vi "TupnOff.vi"(8 "error in (no error)":errorcluster, 11 "Pump_1AI_1DO_2DI in":refnum<class "PM_Group.lvclass">) -> (0 "error out":errorcluster, 3 "Pump_1AI_1DO_2DI out":refnum<class "PM_Group.lvclass">)   [LabVIEW 2019, in "PM_Group.lvclass"]
uses:
  PM_Group.lvclass
  TypeDef/StatePump.ctl
  FPGA_API_class/FPGA API.lvclass
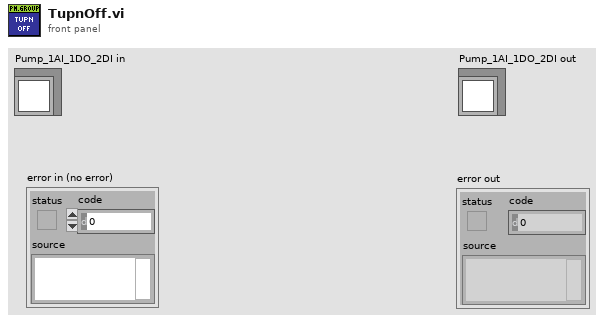
[diagram p1: front panel]
types:
  T1 = typedef "StatePump.ctl" = enum16{"Off", "TupningOn", "On", "TurningOff"}
  T2 = typedef "DO index.ctl" = u8
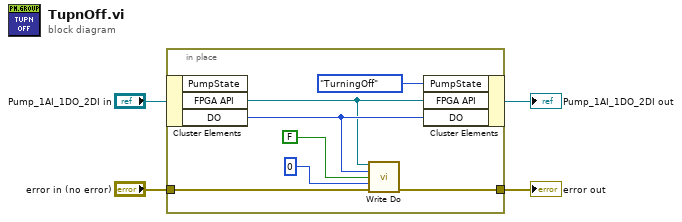
[diagram p0: block diagram]
diagram:
  n1 = in-place {
    in-place-border: "error in (no error)" -> [w7]
    in-place-border: [w6] -> w1
    n2 = in-place-cluster #1("Pump_1AI_1DO_2DI in") -> ("FPGA API"=w5:refnum<class "FPGA API.lvclass">, "DO"=w8:T2)  [unwired: 1 out]
    n3 = call "Write Do.vi"("FPGA API in"=w5, "#DO"=w8, "value"=FALSE, "Time uSec"=u32 0, "error in (no error)"=w7) -> ("error out"=w6:errorcluster)  [unwired: 9 in, 1 out]
    n4 = in-place-cluster #1("PumpState"=StatePump."TurningOff", "FPGA API"=w5, "DO"=w8) -> (→"Pump_1AI_1DO_2DI out":refnum<class "PM_Group.lvclass">)
  }
  "error out" <- w1
